vi "Pre Launch Init.vi"(11 "Acquisition Controller in":refnum<class "Acquisition Controller.lvclass">) -> (0 "error out":errorcluster, 3 "Acquisition Controller out":refnum<class "Acquisition Controller.lvclass">)   [LabVIEW 2016, in "Controllers.lvlib" / "Acquisition Controller.lvclass"]
doc: "(<B>Filename</B>: Actor Framework.lvlib:Actor.lvclass:Pre Launch Init.vi)\n\nDefines behavior that occurs after the Launch Nested Actor method is invoked but before the actor's Actor Core method begins running.\n\nBy default, this method does nothing. A descendant class may override it to define behavior."
uses:
  Acquisition Controller.lvclass
  C:/Program Files (x86)/National Instruments/LabVIEW 2016/vi.lib/ActorFramework/Actor/Actor.lvclass
  Delay Line/DAQmx Delay Line/DAQmx Delay Line.lvclass
  Delay Line/Simulate/Simulate.lvclass
  Photon Counter/C8855/C8855.lvclass
  Photon Counter/Simulate/Simulate.lvclass
  Configurations/Read and Update Key (String).vi
  <vilib>/Utility/error.llb/Error Cluster From Error Code.vi
  <vilib>/ActorFramework/Message Enqueuer/Message Enqueuer.lvclass
  <vilib>/ErrorRing/Error Ring.xnode
  Configurations/Configurations.lvclass
  <vilib>/ActorFramework/Actor/Actor.lvclass
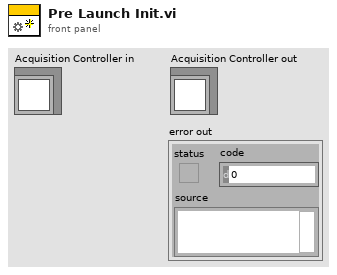
[diagram p1: front panel]
types:
  T1 = typedef "Configurations.lvlib/Configurations.lvclass/Session Handle.ctl" = refnum<data-value>
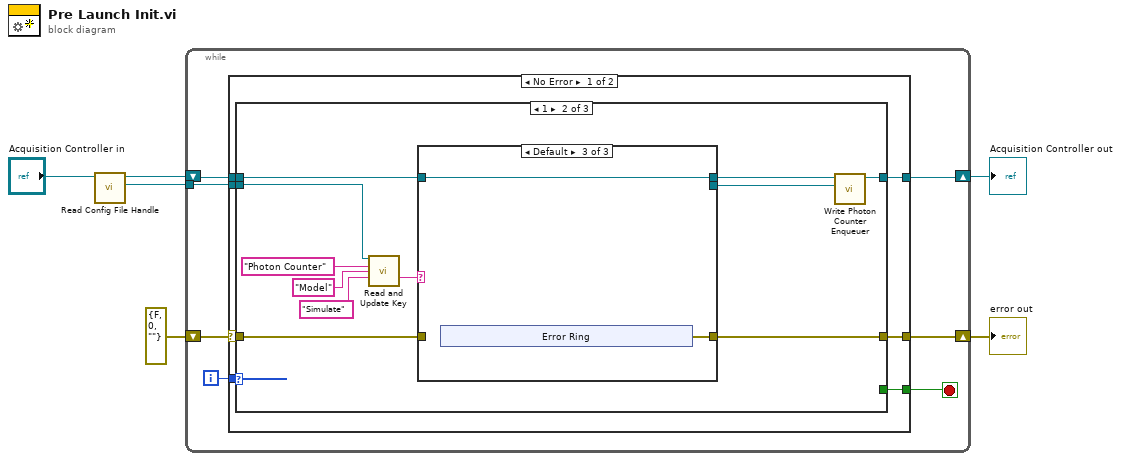
[diagram p0: block diagram]
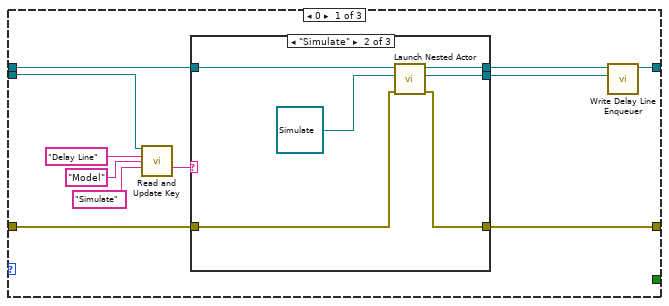
[diagram p2: hidden frame]
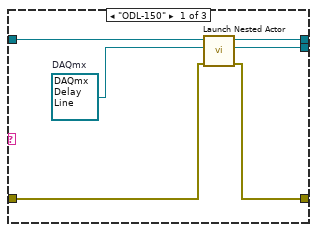
[diagram p3: hidden frame]
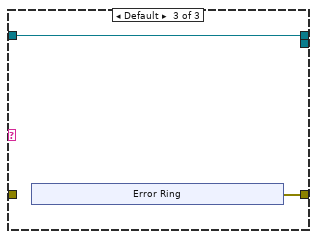
[diagram p4: hidden frame]
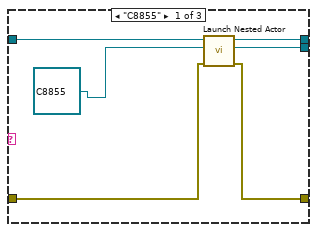
[diagram p5: hidden frame]
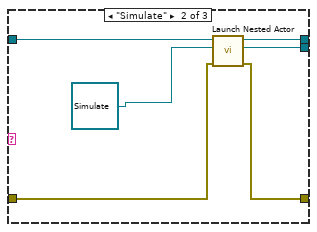
[diagram p6: hidden frame]
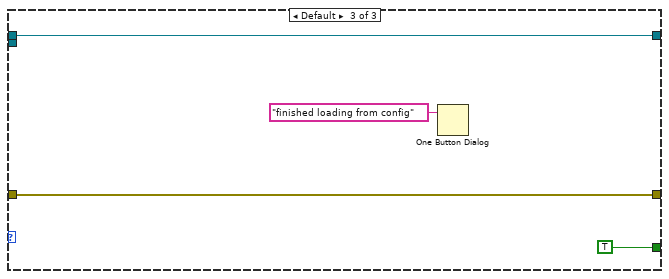
[diagram p7: hidden frame]
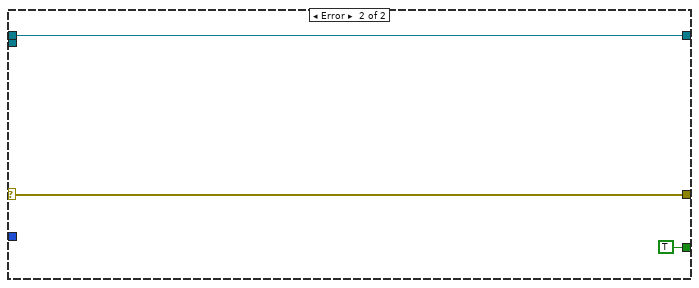
[diagram p8: hidden frame]
diagram:
  n1 = call-dynamic "Read Config File Handle.vi"("Abstract Controller in"="Acquisition Controller in") -> ("Session Handle"=w5:T1, "Abstract Controller out"=w4:refnum<class "Acquisition Controller.lvclass">)  [unwired: 9 in]
  n2 = while {
    tunnel: w5 -> [w13]
    shift-right: [w7] -> w3
    shift-left: w4 -> [w8]
    shift-right: [w10] -> w2
    shift-left: errorcluster {"status"=FALSE, "code"=0, "source"=""} ("error out") -> [w9]
    i -> [w12]
    stop <- w11 stop-if-true
    n3 = case shown="No Error" w9 {
      selector: w9 -> [w16 w85]
      tunnel: w13 -> [w20 _]
      tunnel: w12 -> [w19 _]
      tunnel: [w18 TRUE] -> w11
      tunnel: [w17 w85] -> w10
      tunnel: w8 -> [w15 w83]
      tunnel: [w14 w83] -> w7
      frame No Error {
        n4 = case shown="1" w19 {
          tunnel: w20 -> [w31 w60 _]
          tunnel: [w21 w50 w81] -> w17
          tunnel: [_ _ TRUE] -> w18
          tunnel: w16 -> [w27 w56 w81]
          tunnel: w15 -> [w25 w54 w79]
          tunnel: [w22 w51 w79] -> w14
          frame 0 {
            n5 = call-poly "Read and Update Key.vi"("Session Handle in"=w31, "section"="Delay Line", "key"="Model", "default"="Simulate") -> ("value"=w28:string)  [unwired: 9 in, 2 out]
            n6 = case shown="\"Simulate\"" w28 {
              tunnel: [w34 w38 w45] -> w21
              tunnel: w27 -> [w35 w39 _]
              tunnel: w25 -> [w37 w43 w44]
              tunnel: [w33 w42 w44] -> w24
              tunnel: [w32 w41 _] -> w23
              frame "ODL-150" {
                w36 = refnum<class "DAQmx Delay Line.lvclass"> refnum  # DAQmx
                n7 = call <vilib>:"Launch Nested Actor.vi"("error in (no error)"=w35, "Nested Actor"=w36, "Caller Actor in"=w37) -> ("error out"=w34:errorcluster, "Nested Actor's Enqueuer"=w32:refnum<class "Message Enqueuer.lvclass">, "Caller Actor out"=w33:refnum<class "Acquisition Controller.lvclass">)  [unwired: 6 in]
              }
              frame "Simulate" {
                n8 = call <vilib>:"Launch Nested Actor.vi"("error in (no error)"=w39, "Nested Actor"=refnum<class "Simulate.lvclass"> refnum ("Delay Line.lvlib:Simulate.lvclass"), "Caller Actor in"=w43) -> ("error out"=w38:errorcluster, "Nested Actor's Enqueuer"=w41:refnum<class "Message Enqueuer.lvclass">, "Caller Actor out"=w42:refnum<class "Acquisition Controller.lvclass">)  [unwired: 6 in]
              }
              frame Default {
                n9 = xnode "Error Ring"() -> ("error out"=w45:errorcluster)
              }
            }
            n10 = call-dynamic "Write Delay Line Enqueuer.vi"("Actor Framework:Message Enqueuer"=w23, "Abstract Controller in"=w24) -> ("Abstract Controller out"=w22:refnum<class "Acquisition Controller.lvclass">)  [unwired: 9 in]
          }
          frame 1 {
            n11 = call-poly "Read and Update Key.vi"("Session Handle in"=w60, "section"="Photon Counter", "key"="Model", "default"="Simulate") -> ("value"=w57:string)  [unwired: 9 in, 2 out]
            n12 = case shown="Default" w57 {
              tunnel: [w64 w68 w74] -> w50
              tunnel: w56 -> [w65 w69 _]
              tunnel: w54 -> [w66 w72 w73]
              tunnel: [w63 w71 w73] -> w53
              tunnel: [w62 w70 _] -> w52
              frame "C8855" {
                n13 = call <vilib>:"Launch Nested Actor.vi"("error in (no error)"=w65, "Nested Actor"=refnum<class "C8855.lvclass"> refnum ("Photon Counter.lvlib:C8855.lvclass"), "Caller Actor in"=w66) -> ("error out"=w64:errorcluster, "Nested Actor's Enqueuer"=w62:refnum<class "Message Enqueuer.lvclass">, "Caller Actor out"=w63:refnum<class "Acquisition Controller.lvclass">)  [unwired: 6 in]
              }
              frame "Simulate" {
                n14 = call <vilib>:"Launch Nested Actor.vi"("error in (no error)"=w69, "Nested Actor"=refnum<class "Simulate.lvclass"> refnum ("Photon Counter.lvlib:Simulate.lvclass"), "Caller Actor in"=w72) -> ("error out"=w68:errorcluster, "Nested Actor's Enqueuer"=w70:refnum<class "Message Enqueuer.lvclass">, "Caller Actor out"=w71:refnum<class "Acquisition Controller.lvclass">)  [unwired: 6 in]
              }
              frame Default {
                n15 = xnode "Error Ring"() -> ("error out"=w74:errorcluster)
              }
            }
            n16 = call-dynamic "Write Photon Counter Enqueuer.vi"("Actor Framework:Message Enqueuer"=w52, "Abstract Controller in"=w53) -> ("Abstract Controller out"=w51:refnum<class "Acquisition Controller.lvclass">)  [unwired: 9 in]
          }
          frame Default {
            n17 = One Button Dialog(message="finished loading from config") -> ()  [unwired: 1 in, 1 out]
          }
        }
      }
      frame Error {
      }
    }
  }
  "error out" <- w2
  "Acquisition Controller out" <- w3
